vi "Math-Discrete Truncated Exponential RNG.vi"(0 "samples":i32, 5 "Min":dbl, 7 "Max":dbl, 9 "Step":dbl, 11 "Lambda":dbl) -> (4 "Array":dbl[](array[numeric]))   [LabVIEW 2020]
uses:
  LinSpace (start-stop-step).vi
  <vilib>/Analysis/NI_AALPro.lvlib
panel:
  out "Histogram":T1(graph)
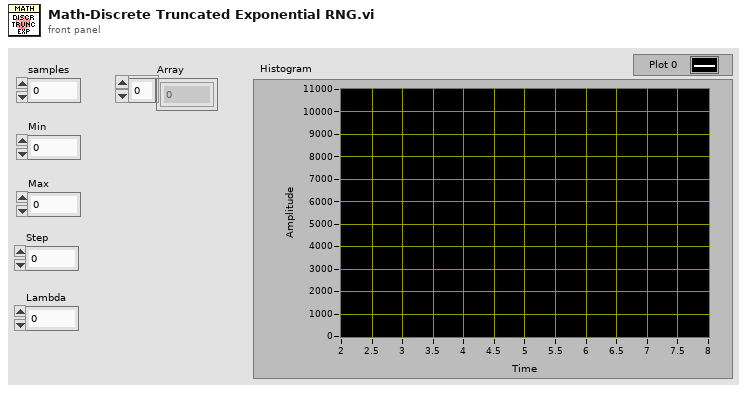
[diagram p1: front panel]
types:
  T1 = cluster{"X Values":dbl[], "Histogram: h(x)":i32[]}
  T2 = cluster{dbl, dbl, "inclusion":enum32{"lower", "upper"}}
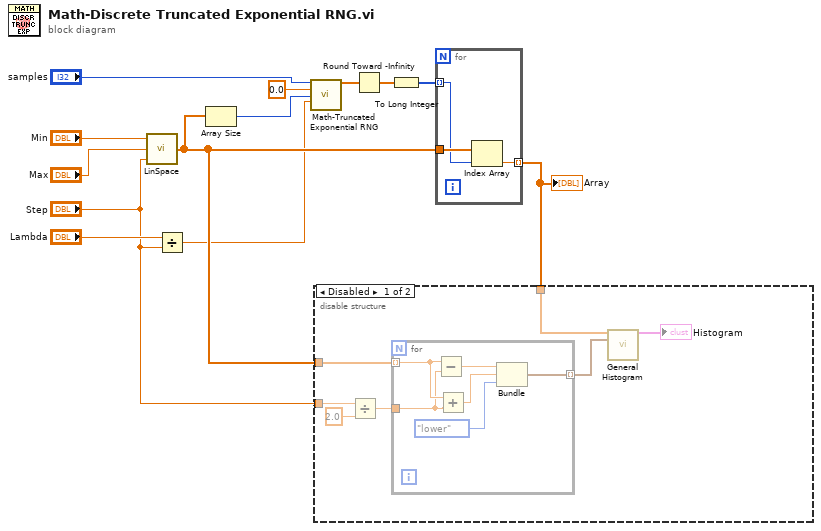
[diagram p0: block diagram]
diagram:
  n1 = call-poly "LinSpace.vi"("Step"="Step", "Stop"="Max", "Start"="Min") -> ("Array"=w3:dbl[])  [unwired: 1 in, 1 out]
  n2 = Divide(x="Lambda", y="Step") -> (x/y=w2:dbl)
  n3 = Array Size(array=w3) -> (size(s)=w4:i32)
  n4 = call "Math-Truncated Exponential RNG.vi"("samples"="samples", "Min"=0.0, "Max"=w4, "Lambda"=w2) -> ("Array"=w10:dbl[])  [unwired: 11 in]
  n5 = Round Toward -Infinity(1:w10) -> (0:w9:dbl[])
  n6 = To Long Integer(number=w9) -> (32bit integer=w8:i32[])
  n7 = for {
    tunnel: w8 -> [w15] mode=indexing
    tunnel: w3 -> [w16]
    tunnel: [w14] -> w7 mode=indexing
    n8 = Index Array(array=w16, index=w15) -> (element=w14:dbl)
  }
  "Array" <- w7
  n9 = disable-structure shown="Disabled" {
    disable-tunnel: w7 -> [w23 _]
    disable-tunnel: w3 -> [w22 _]
    disable-tunnel: "Step" -> [w18 _]
    frame Disabled {
      n10 = Divide(x=w18, y=2.0) -> (x/y=w20:dbl)
      n11 = for {
        tunnel: w22 -> [w29] mode=indexing
        tunnel: w20 -> [w28]
        tunnel: [w24] -> w19 mode=indexing
        n12 = Subtract(x=w29, y=w28) -> (x-y=w27:dbl)
        n13 = Add(x=w29, y=w28) -> (x+y=w26:dbl)
        n14 = Bundle(w27, w26, "inclusion"=enum32{"lower", "upper"}."lower") -> (w24:T2)  [unwired: 1 in]
      }
      n15 = call <vilib>:"General Histogram.vi"("X"=w23, "Bins"=w19) -> ("Histogram Graph"=→"Histogram":T1)  [unwired: 9 in, 4 out]
    }
    frame Enabled {
    }
  }
